vi "DB_LeePower_Graficas.vi"(8 "error in (no error)":errorcluster, 11 "ID_EQUIPO":i32=1) -> (0 "error out":errorcluster, 3 "Power out":T1)   [LabVIEW 2018]
uses:
  Controls/Power_cluster.ctl
  <vilib>/addons/database/Connection.llb/DB Tools Open Connec (Path).vi
  <vilib>/addons/database/Connection.llb/Conn Execute.vi
  <vilib>/addons/database/Recordset.llb/Rec Fetch Recordset Data (R).vi
  <vilib>/addons/database/Recordset.llb/Rec Destroy - Connection.vi
  <vilib>/addons/database/_DB Variant To Data/Database Variant To Data.xnode
  <vilib>/addons/database/NI_Database_API.lvlib
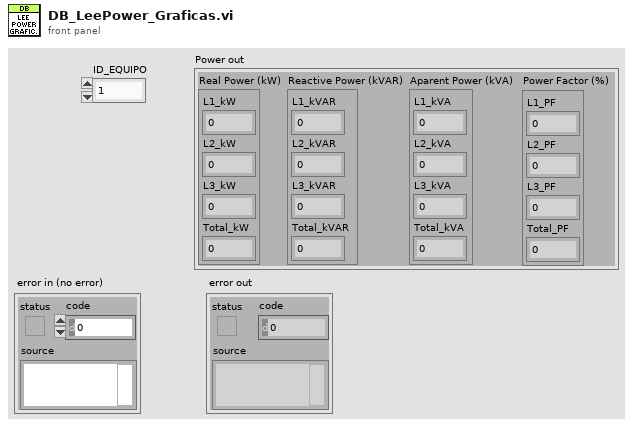
[diagram p1: front panel]
types:
  T1 = typedef "Power_cluster.ctl" = cluster{"Real Power (kW)":cluster{"L1_kW":sgl, "L2_kW":sgl, "L3_kW":sgl, "Total_kW":sgl}, "Reactive Power (kVAR)":cluster{"L1_kVAR":sgl, "L2_kVAR":sgl, "L3_kVAR":sgl, "Total_kVAR":sgl}, "Aparent Power (kVA)":cluster{"L1_kVA":sgl, "L2_kVA":sgl, "L3_kVA":sgl, "Total_kVA":sgl}, "Power Factor (%)":cluster{"L1_PF":sgl, "L2_PF":sgl, "L3_PF":sgl, "Total_PF":sgl}}
  T2 = cluster{"L1_PF":sgl, "L2_PF":sgl, "L3_PF":sgl, "Total_PF":sgl}
  T3 = cluster{"L1_kVA":sgl, "L2_kVA":sgl, "L3_kVA":sgl, "Total_kVA":sgl}
  T4 = cluster{"L1_kVAR":sgl, "L2_kVAR":sgl, "L3_kVAR":sgl, "Total_kVAR":sgl}
  T5 = cluster{"L1_kW":sgl, "L2_kW":sgl, "L3_kW":sgl, "Total_kW":sgl}
  T6 = typedef "NI_Database_API.lvlib/Conn ObjectReference.ctl" = refnum<k1>
  T7 = typedef "NI_Database_API.lvlib/Rec ObjectReference.ctl" = refnum<k1>
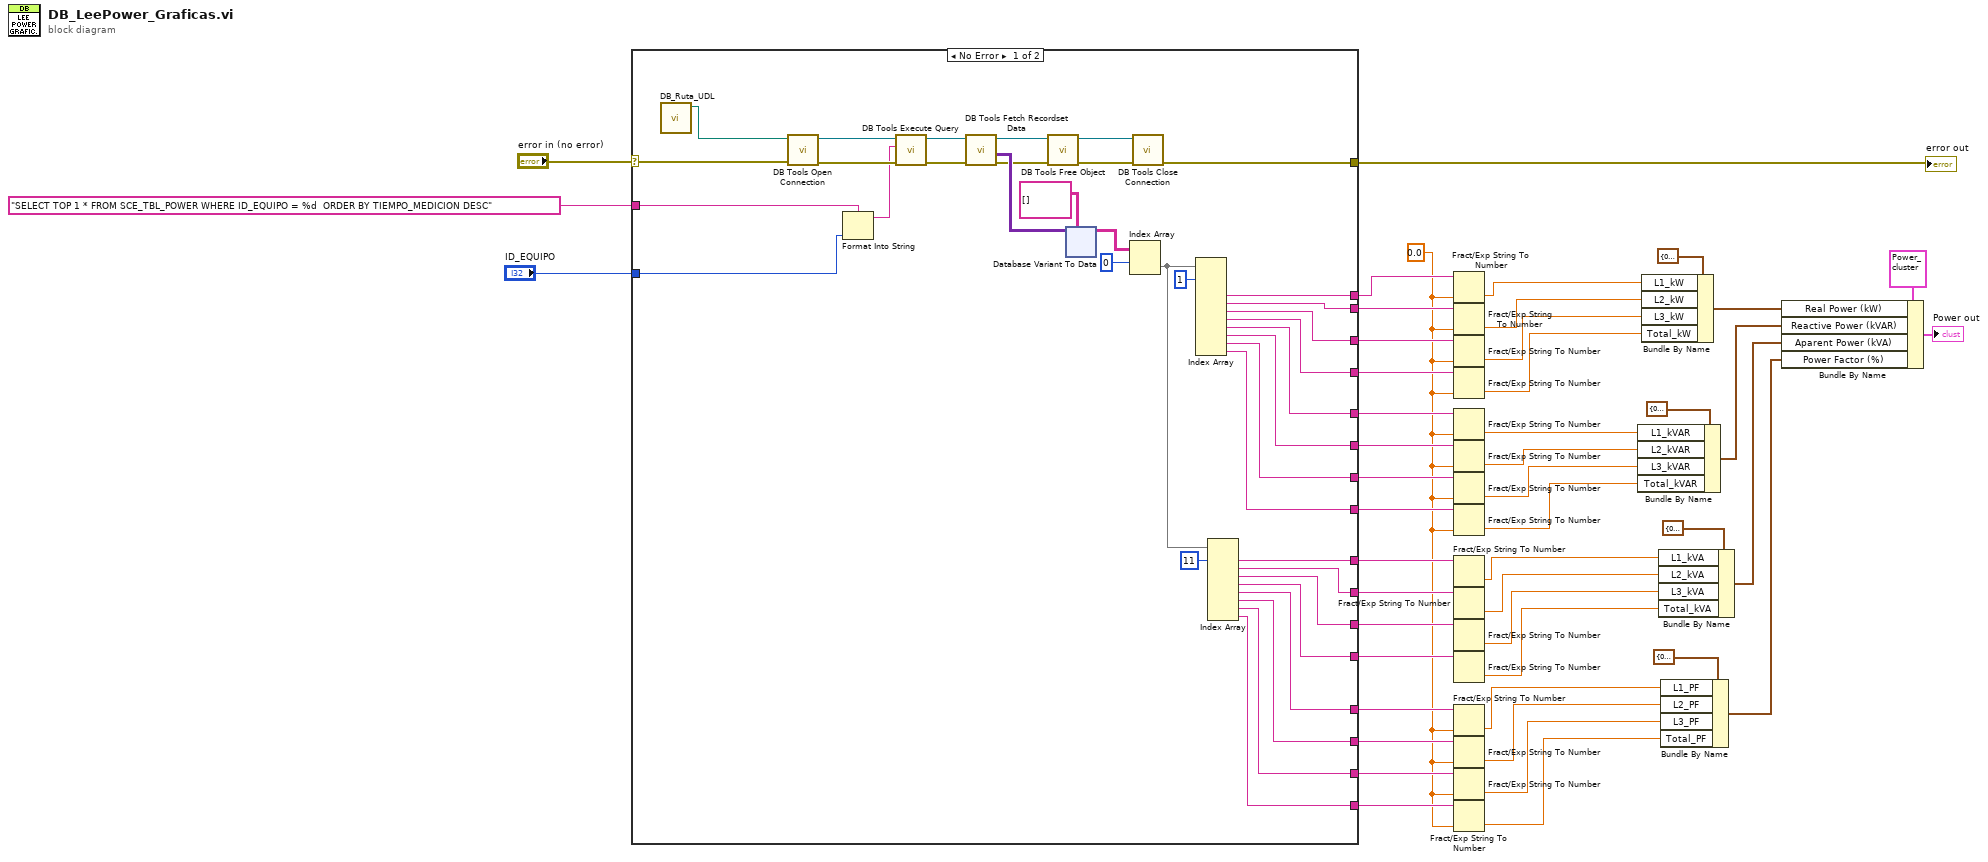
[diagram p0: block diagram]
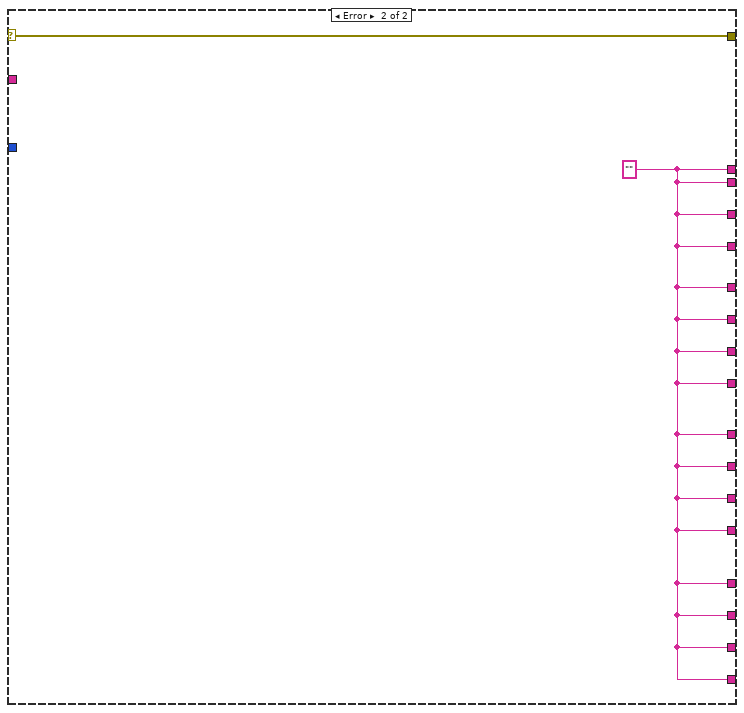
[diagram p2: hidden frame]
diagram:
  w9 = sgl 0.0
  n1 = case shown="No Error" "error in (no error)" {
    selector: "error in (no error)" -> [w79 w130]
    tunnel: [w81 w130] -> w45
    tunnel: "SELECT TOP 1 * FROM SCE_TBL_POWER WHERE ID_EQUIPO = %d  ORDER BY TIEMPO_MEDICION DESC" ("SQL") -> [w71 _]
    tunnel: [w68 w129] -> w43
    tunnel: [w67 w129] -> w42
    tunnel: [w66 w129] -> w41
    tunnel: "ID_EQUIPO" -> [w69 _]
    tunnel: [w64 w129] -> w40
    tunnel: [w65 w129] -> w39
    tunnel: [w63 w129] -> w38
    tunnel: [w61 w129] -> w29
    tunnel: [w60 w129] -> w28
    tunnel: [w57 w129] -> w17
    tunnel: [w56 w129] -> w16
    tunnel: [w55 w129] -> w15
    tunnel: [w54 w129] -> w14
    tunnel: [w53 w129] -> w13
    tunnel: [w52 w129] -> w12
    tunnel: [w51 w129] -> w11
    tunnel: [w50 w129] -> w10
    frame No Error {
      n2 = call "DB_Ruta_UDL.vi"() -> ("UDL ruta"=w49:path)  [unwired: 11 in]
      n3 = call-poly <vilib>:"DB Tools Open Connection.vi"("error in (no error)"=w79, "connection information"=w49) -> ("error out"=w84:errorcluster, "connection reference"=w82:T6)  [unwired: 6 in]
      n4 = Format Into String(format string=w71, w69) -> (resulting string=w70:string)  [unwired: 2 in, 1 out]
      n5 = call-poly <vilib>:"DB Tools Execute Query.vi"("error in (no error)"=w84, "SQL query"=w70, "connection reference"=w82) -> ("error out"=w80:errorcluster, "recordset reference"=w78:T7)  [unwired: 5 in]
      n6 = call-poly <vilib>:"DB Tools Fetch Recordset Data.vi"("error in (no error)"=w80, "recordset reference"=w78) -> ("error out"=w74:errorcluster, "recordset data"=w75:variant[][], "recordset reference out"=w77:T7)  [unwired: 3 in]
      n7 = call-poly <vilib>:"DB Tools Free Object.vi"("error in (no error)"=w74, "recordset reference"=w77) -> ("error out"=w83:errorcluster, "connection reference"=w48:T6)  [unwired: 8 in]
      n8 = xnode "Database Variant To Data"("database variant"=w75, "type"=string[][] []) -> ("data"=w73:string[][])  [unwired: 1 in, 1 out]
      n9 = Index Array(array=w73, index (row)=0 ("disabled index (col)")) -> (element=w58:string[])  [unwired: 1 in]
      n10 = call <vilib>:"DB Tools Close Connection.vi"("error in (no error)"=w83, "connection reference"=w48) -> ("error out"=w81:errorcluster)  [unwired: 5 in]
      n11 = Index Array(array=w58, index #1=1 ("index")) -> (element #3=w68:string, element #4=w67:string, element #5=w66:string, element #6=w61:string, element #7=w64:string, element #8=w65:string, element #9=w63:string, element #10=w60:string)  [unwired: 9 in, 2 out]
      n12 = Index Array(array=w58, index #1=11 ("index")) -> (element #1=w57:string, element #2=w56:string, element #3=w55:string, element #4=w54:string, element #5=w53:string, element #6=w52:string, element #7=w51:string, element #8=w50:string)  [unwired: 7 in]
    }
    frame Error {
      w129 = ""
    }
  }
  "error out" <- w45
  n13 = Fract/Exp String To Number(string=w43, default (0 dbl)=w9) -> (number=w36:sgl)  [unwired: 2 in, 1 out]
  n14 = Fract/Exp String To Number(string=w42, default (0 dbl)=w9) -> (number=w35:sgl)  [unwired: 2 in, 1 out]
  n15 = Fract/Exp String To Number(string=w41, default (0 dbl)=w9) -> (number=w34:sgl)  [unwired: 2 in, 1 out]
  n16 = Fract/Exp String To Number(string=w29, default (0 dbl)=w9) -> (number=w26:sgl)  [unwired: 2 in, 1 out]
  n17 = Fract/Exp String To Number(string=w40, default (0 dbl)=w9) -> (number=w33:sgl)  [unwired: 2 in, 1 out]
  n18 = Fract/Exp String To Number(string=w39, default (0 dbl)=w9) -> (number=w32:sgl)  [unwired: 2 in, 1 out]
  n19 = Fract/Exp String To Number(string=w38, default (0 dbl)=w9) -> (number=w31:sgl)  [unwired: 2 in, 1 out]
  n20 = Fract/Exp String To Number(string=w28, default (0 dbl)=w9) -> (number=w27:sgl)  [unwired: 2 in, 1 out]
  n21 = Fract/Exp String To Number(string=w17) -> (number=w8:dbl)  [unwired: 3 in, 1 out]
  n22 = Fract/Exp String To Number(string=w16) -> (number=w7:dbl)  [unwired: 3 in, 1 out]
  n23 = Fract/Exp String To Number(string=w15) -> (number=w6:dbl)  [unwired: 3 in, 1 out]
  n24 = Fract/Exp String To Number(string=w14) -> (number=w5:dbl)  [unwired: 3 in, 1 out]
  n25 = Fract/Exp String To Number(string=w13, default (0 dbl)=w9) -> (number=w4:sgl)  [unwired: 2 in, 1 out]
  n26 = Fract/Exp String To Number(string=w12, default (0 dbl)=w9) -> (number=w3:sgl)  [unwired: 2 in, 1 out]
  n27 = Fract/Exp String To Number(string=w11, default (0 dbl)=w9) -> (number=w2:sgl)  [unwired: 2 in, 1 out]
  n28 = Fract/Exp String To Number(string=w10, default (0 dbl)=w9) -> (number=w1:sgl)  [unwired: 2 in, 1 out]
  n29 = Bundle By Name(cluster=T4 {"L1_kVAR"=0.0, "L2_kVAR"=0.0, "L3_kVAR"=0.0, "Total_kVAR"=0.0} ("Reactive Power (kVAR)"), "L1_kVAR"=w33, "L2_kVAR"=w32, "L3_kVAR"=w31, "Total_kVAR"=w27) -> (w30:T4)
  n30 = Bundle By Name(cluster=T5 {"L1_kW"=0.0, "L2_kW"=0.0, "L3_kW"=0.0, "Total_kW"=0.0} ("Real Power (kW)"), "L1_kW"=w36, "L2_kW"=w35, "L3_kW"=w34, "Total_kW"=w26) -> (w37:T5)
  n31 = Bundle By Name(cluster=T3 {"L1_kVA"=0.0, "L2_kVA"=0.0, "L3_kVA"=0.0, "Total_kVA"=0.0} ("Aparent Power (kVA)"), "L1_kVA"=w8, "L2_kVA"=w7, "L3_kVA"=w6, "Total_kVA"=w5) -> (w20:T3)
  n32 = Bundle By Name(cluster=T2 {"L1_PF"=0.0, "L2_PF"=0.0, "L3_PF"=0.0, "Total_PF"=0.0} ("Power Factor (%)"), "L1_PF"=w4, "L2_PF"=w3, "L3_PF"=w2, "Total_PF"=w1) -> (w19:T2)
  n33 = Bundle By Name(cluster=T1 {"Real Power (kW)"={"L1_kW"=0.0, "L2_kW"=0.0, "L3_kW"=0.0, "Total_kW"=0.0}, "Reactive Power (kVAR)"={"L1_kVAR"=0.0, "L2_kVAR"=0.0, "L3_kVAR"=0.0, "Total_kVAR"=0.0}, "Aparent Power (kVA)"={"L1_kVA"=0.0, "L2_kVA"=0.0, "L3_kVA"=0.0, "Total_kVA"=0.0}, "Power Factor (%)"={"L1_PF"=0.0, "L2_PF"=0.0, "L3_PF"=0.0, "Total_PF"=0.0}} ("Power_cluster"), "Real Power (kW)"=w37, "Reactive Power (kVAR)"=w30, "Aparent Power (kVA)"=w20, "Power Factor (%)"=w19) -> (→"Power out":T1)
